vi "Self-Test.vi"(0 "VISA resource name":refnum<visa-resource-name>, 11 "error in (no error)":errorcluster) -> (4 "VISA resource name out":refnum<visa-resource-name>, 8 "Self-Test Result Code":u32, 10 "Self-Test Result Message":string, 15 "error out":errorcluster)   [LabVIEW 2020, in "Keithley 27XX.lvlib"]
doc: "This VI causes the instrument to perform a self-test and returns the results. A numeric indicator indicates if the instrument passed all self-tests, and a string indicator contains the instrument's reponse.\n\nNote: This VI is only supported across GPIB."
uses:
  Keithley 27XX.lvlib
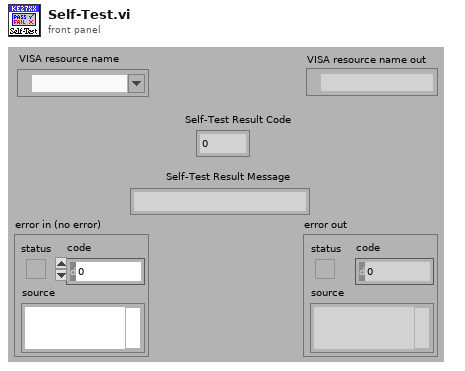
[diagram p1: front panel]
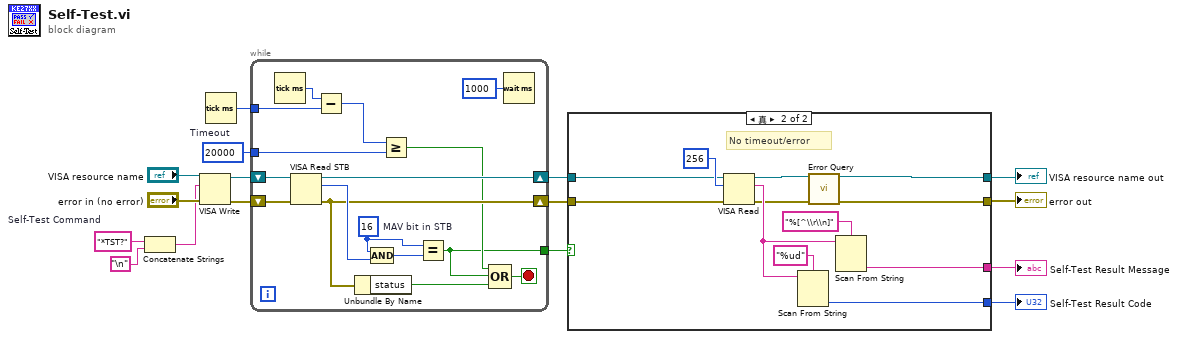
[diagram p0: block diagram]
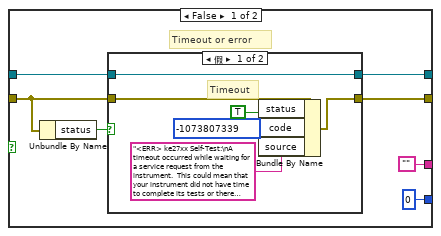
[diagram p2: hidden frame]
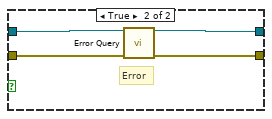
[diagram p3: hidden frame]
diagram:
  w13 = u32 20000  # Timeout
  w3 = "*TST?"  # Self-Test Command
  n1 = Concatenate Strings(w3, "\n") -> (w1:string)
  n2 = VISA Write(VISA resource name="VISA resource name", write buffer=w1, error in (no error)="error in (no error)") -> (VISA resource name out=w16:refnum<visa-resource-name>, error out=w15:errorcluster)  [unwired: 1 out]
  n3 = Tick Count (ms)() -> (millisecond timer value=w14:u32)
  n4 = while {
    shift-right: [w25] -> w9
    shift-left: w15 -> [w29]
    shift-right: [w27] -> w10
    shift-left: w16 -> [w28]
    tunnel: w14 -> [w21]
    tunnel: w13 -> [w19]
    tunnel: [w17] -> w4
    stop <- w23 stop-if-true
    w32 = u16 16  # MAV bit in STB
    n5 = Tick Count (ms)() -> (millisecond timer value=w22:u32)
    n6 = VISA Read STB(8:w29, 11:w28) -> (0:w25:errorcluster, 2:w30:u16, 3:w27:refnum<visa-resource-name>)
    n7 = Subtract(x=w22, y=w21) -> (x-y=w20:u32)
    n8 = Unbundle By Name(w25) -> ("status"=w24:bool)
    n9 = Compound Arithmetic op=AND(w32, w30) -> (w31:u16)
    n10 = Greater Or Equal?(x=w20, y=w19) -> (x >= y?=w18:bool)
    n11 = Equal?(x=w32, y=w31) -> (x = y?=w17:bool)
    n12 = Compound Arithmetic op=OR(w18, w17, w24) -> (w23:bool)
    n13 = Wait (ms)(milliseconds to wait=u32 1000) -> ()  [unwired: 1 out]
  }
  n14 = case shown="真" w4 {
    tunnel: ["" w61] -> w6
    tunnel: w10 -> [w38 w58]
    tunnel: w9 -> [w36 w57]
    tunnel: [0 w54] -> w5
    tunnel: [w37 w51] -> w8
    tunnel: [w35 w50] -> w7
    frame False {
      # "Timeout or error"
      n15 = Unbundle By Name(w36) -> ("status"=w39:bool)
      n16 = case shown="假" w39 {
        tunnel: w38 -> [w40 w49]
        tunnel: [w40 w46] -> w37
        tunnel: [w41 w47] -> w35
        tunnel: w36 -> [w42 w48]
        frame False {
          # "Timeout"
          n17 = Bundle By Name(cluster=w42, "status"=TRUE, "code"=-1073807339, "source"="<ERR> ke27xx Self-Test:\nA timeout occurred while waiting for a service request from the instrument.  This could mean that your instrument did not have time to complete its tests or there could be a problem communicating with the instrument.") -> (w41:errorcluster)
        }
        frame True {
          # "Error"
          n18 = call "Error Query.vi"("VISA resource name"=w49, "error in (no error)"=w48) -> ("VISA resource name out"=w46:refnum<visa-resource-name>, "error out"=w47:errorcluster)  [unwired: 10 in, 2 out]
        }
      }
    }
    frame True {
      # "No timeout/error"
      n19 = VISA Read(VISA resource name=w58, byte count=u32 256, error in (no error)=w57) -> (VISA resource name out=w52:refnum<visa-resource-name>, read buffer=w56:string, error out=w53:errorcluster)  [unwired: 1 out]
      n20 = Scan From String(format string="%ud", input string=w56) -> (output 1=w54:u32)  [unwired: 3 in, 3 out]
      n21 = call "Error Query.vi"("VISA resource name"=w52, "error in (no error)"=w53) -> ("VISA resource name out"=w51:refnum<visa-resource-name>, "error out"=w50:errorcluster)  [unwired: 10 in, 2 out]
      n22 = Scan From String(format string="%[^\\r\\n]", input string=w56) -> (output 1=w61:string)  [unwired: 3 in, 3 out]
    }
  }
  "Self-Test Result Message" <- w6
  "Self-Test Result Code" <- w5
  "error out" <- w7
  "VISA resource name out" <- w8
